vi "ViewQueue.vi"(5 "Image queue":refnum<queue>) -> (1 "Slider Indexes":cluster{i16, i16, i16}={1, 46, 100}, 2 "Save?":bool)   [LabVIEW 2022 SP3]
uses:
  <vilib>/picture/picture.llb/imagedata.ctl
panel:
  out "Display Image":i32
  in  "Save Image\nRange":bool
  in  "ExitSendCmd":bool
  out "2D Picture":picture
  in  "Element":cluster{i16, i16, i16}(slide)={1, 40, 100} scale=1.0..100.0
  # "Middle slider is visible image. Low and high select the range to save."
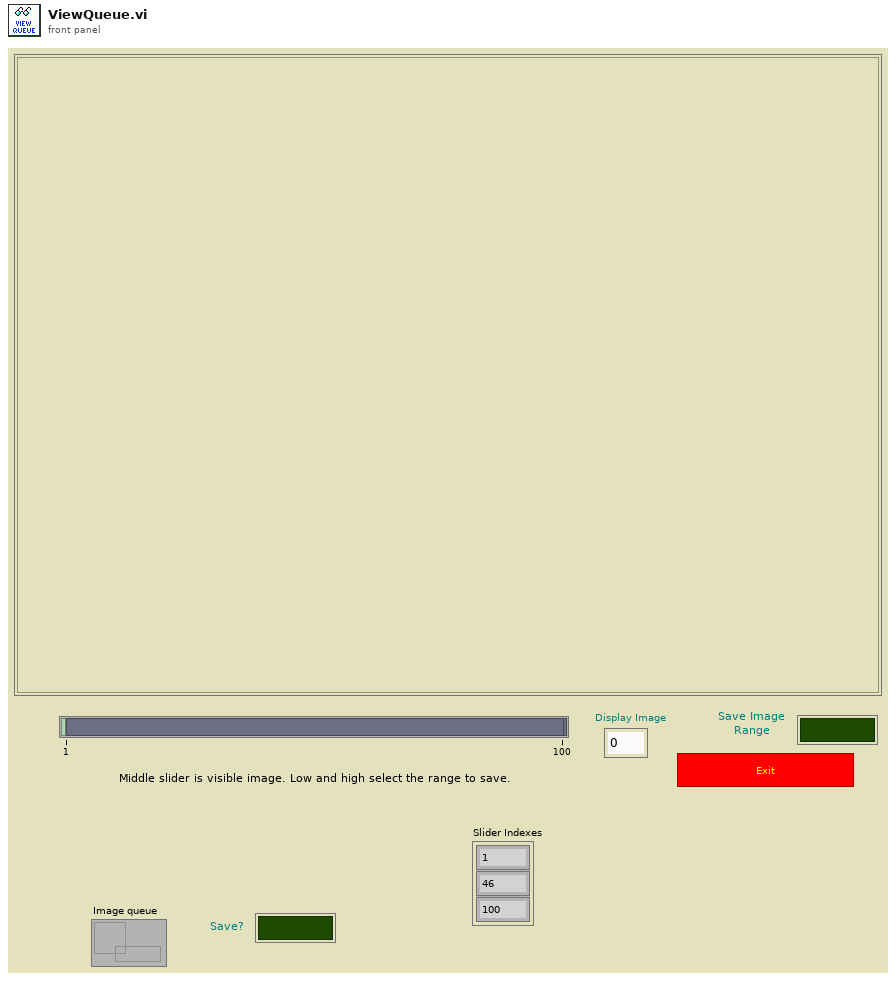
[diagram p1: front panel]
types:
  T1 = typedef "imagedata.ctl" = cluster{"image type":i32, "image depth":i32, "image":u8[], "mask":u8[], "colors":u32[], "Rectangle":cluster{"left":i16, "top":i16, "right":i16, "bottom":i16}}
  T2 = cluster{"N":u8, "N":u8, "# elements in queue":i32}
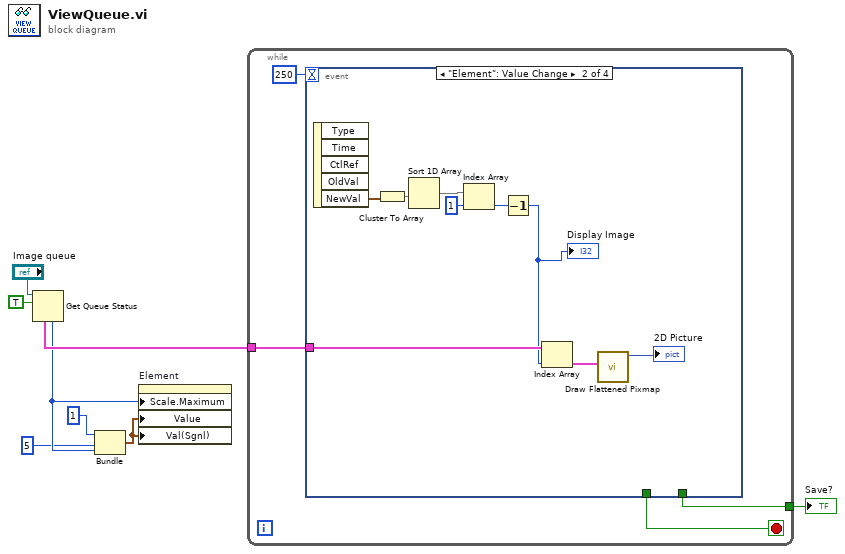
[diagram p0: block diagram]
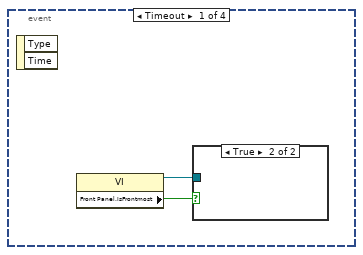
[diagram p2: hidden frame]
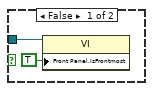
[diagram p3: hidden frame]
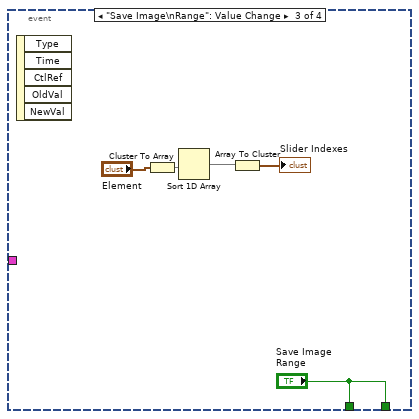
[diagram p4: hidden frame]
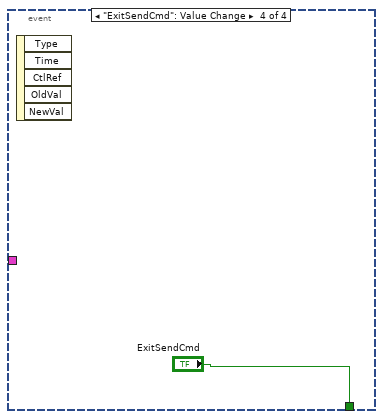
[diagram p5: hidden frame]
diagram:
  n1 = Get Queue Status(queue="Image queue", return elements? (F)=TRUE) -> (# elements in queue=w4:i32, elements=w7:T1[])  [unwired: 1 in, 6 out]
  n2 = Bundle("N"=u8 1, "N"=u8 5, "# elements in queue"=w4) -> (w1:T2)  [unwired: 1 in]
  n3 = property on="Element" class="Slide (strict)"("Scale.Maximum"=w4, "Value"=w1, "Val(Sgnl)"=w1) -> ()  [unwired: 2 in, 2 out]
  n4 = while {
    tunnel: w7 -> [w12]
    tunnel: [w9] -> w5
    stop <- w10 stop-if-true
    n5 = event shown="[1] \"Element\": Value Change" {
      selector: _ -> [_ _ _ _]
      dyn-events: _ -> [_ _ _ _]
      timeout: 250 -> [_ _ _ _]
      tunnel: w12 -> [_ w25 _ _]
      tunnel: [_ _ "Save Image\nRange" "ExitSendCmd"] -> w10
      tunnel: [_ _ "Save Image\nRange" _] -> w9
      event Timeout {
        n6 = event-data() -> ()  [unwired: 1 in, 2 out]
        n7 = property class="VI"() -> (reference out=w13:refnum<vi>, "Front Panel.IsFrontmost"=w14:bool)  [unwired: 2 in, 1 out]
        n8 = case shown="True" w14 {
          tunnel: w13 -> [w15 _]
          frame False {
            n9 = property class="VI"(reference=w15, "Front Panel.IsFrontmost"=TRUE ("Front Panel Window:Is Frontmost")) -> ()  [unwired: 1 in, 2 out]
          }
          frame True {
          }
        }
      }
      event "Element": Value Change {
        n10 = event-data() -> ("NewVal"=w22:cluster{i16, i16, i16})  [unwired: 1 in, 4 out]
        n11 = Cluster To Array(cluster=w22) -> (array=w21:i16[])
        n12 = Sort 1D Array(array=w21) -> (sorted array=w20:i16[])
        n13 = Index Array(array=w20, index=1) -> (element=w18:i16)
        n14 = Decrement(x=w18) -> (x-1=w17:i16)
        "Display Image" <- w17
        n15 = Index Array(array=w25, index=w17) -> (element=w24:T1)
        n16 = call <vilib>:"Draw Flattened Pixmap.vi"("image data"=w24) -> ("new picture"=→"2D Picture":picture)  [unwired: 8 in]
      }
      event "Save Image\nRange": Value Change {
        n17 = event-data() -> ()  [unwired: 1 in, 5 out]
        n18 = Cluster To Array(cluster="Element") -> (array=w29:i16[])
        n19 = Sort 1D Array(array=w29) -> (sorted array=w27:i16[])
        n20 = Array To Cluster(array=w27) -> (cluster=→"Slider Indexes":cluster{"[0]":i16, "[1]":i16, "[2]":i16})
      }
      event "ExitSendCmd": Value Change {
        n21 = event-data() -> ()  [unwired: 1 in, 5 out]
      }
    }
  }
  "Save?" <- w5
